vi "Initialize.vi"(8 "error in (no error)":errorcluster, 11 "State in":T1={"State"=enum."Idle", "Start Time"=timestamp(0 s since 1904-01-01), "Configuration"={"Cycle Period"=0.0, "Setpoint Entry"=0.0, "Output Device"=enum."Huber Ministat 230", "Huber Ministat 230 Settings"={"VISA resource name"="", "Simulated?"=FALSE}, "Lauda Settings"={"VISA resource name"="", "Simulated?"=FALSE, "Pump Power"=2}, "Julabo FP-50 Settings"={"VISA resource name"="", "Simulated?"=FALSE, "Pump Power"=2}, "Internal Control?"=FALSE, "Huber Unistat 410 Settings"={"VISA resource name"="", "Address"=0, "Simulated?"=FALSE}}, "Current Time"=timestamp(0 s since 1904-01-01), "First Iteration"=FALSE, "Data"={"TCU Speed"=0.0, "Temperature"=0.0}, "Process Name"="", "TCU On?"=FALSE, "Output Error"=FALSE, "Start Log"=FALSE, "Power Level Changed"=FALSE} {"Configuration"."Huber Unistat 410 Settings"."Address" min=0 max=99 format="%02.0f"; "Configuration"."Julabo FP-50 Settings"."Pump Power" min=0 max=8 step=1; "Configuration"."Lauda Settings"."Pump Power" min=0 max=8 step=1}) -> (0 "error out":errorcluster, 3 "State out":T1={"State"=enum."Idle", "Start Time"=timestamp(0 s since 1904-01-01), "Configuration"={"Cycle Period"=0.0, "Setpoint Entry"=0.0, "Output Device"=enum."Huber Ministat 230", "Huber Ministat 230 Settings"={"VISA resource name"="", "Simulated?"=FALSE}, "Lauda Settings"={"VISA resource name"="", "Simulated?"=FALSE, "Pump Power"=2}, "Julabo FP-50 Settings"={"VISA resource name"="", "Simulated?"=FALSE, "Pump Power"=2}, "Internal Control?"=FALSE, "Huber Unistat 410 Settings"={"VISA resource name"="", "Address"=0, "Simulated?"=FALSE}}, "Current Time"=timestamp(0 s since 1904-01-01), "First Iteration"=FALSE, "Data"={"TCU Speed"=0.0, "Temperature"=0.0}, "Process Name"="", "TCU On?"=FALSE, "Output Error"=FALSE, "Start Log"=FALSE, "Power Level Changed"=FALSE} {"Configuration"."Huber Unistat 410 Settings"."Address" min=0 max=99 format="%02.0f"; "Configuration"."Julabo FP-50 Settings"."Pump Power" min=0 max=8 step=1; "Configuration"."Lauda Settings"."Pump Power" min=0 max=8 step=1})   [LabVIEW 2018, in "TCU Module.lvlib" / "TCU Module Engine.lvlib"]
uses:
  TCU Module Engine.lvlib
  TCU State Cluster.ctl
  State Enum.ctl
  TCU Module Settings Cluster.ctl
  Output Devices.ctl
  Huber TCU/Huber Settings.ctl
  Lauda Integral XT-150 TCU/Lauda Settings.ctl
  Julabo Type 1 TCU/Julabo Type 1 TCU Folder/Julabo FP-50 Settings.ctl
  Huber Unistat 410 TCU/Huber Unistat 410 RS485 Settings.ctl
  Tag VIs/Tag FGV Operation Enum.ctl
  Shared Variables/Dynamic Shared Variables.lvlib
  Huber TCU/Huber Ministat 230 TCU.lvlib
  Lauda Integral XT-150 TCU/Lauda TCU.lvlib
  Julabo Type 1 TCU/Julabo Type 1 TCU Folder/Julabo Type FP-50 TCU.lvlib
  Huber Unistat 410 TCU/Huber Unistat 410 TCU.lvlib
  TCU Module.lvlib
panel:
  # "Output Instruments"
  # "Output Instruments"
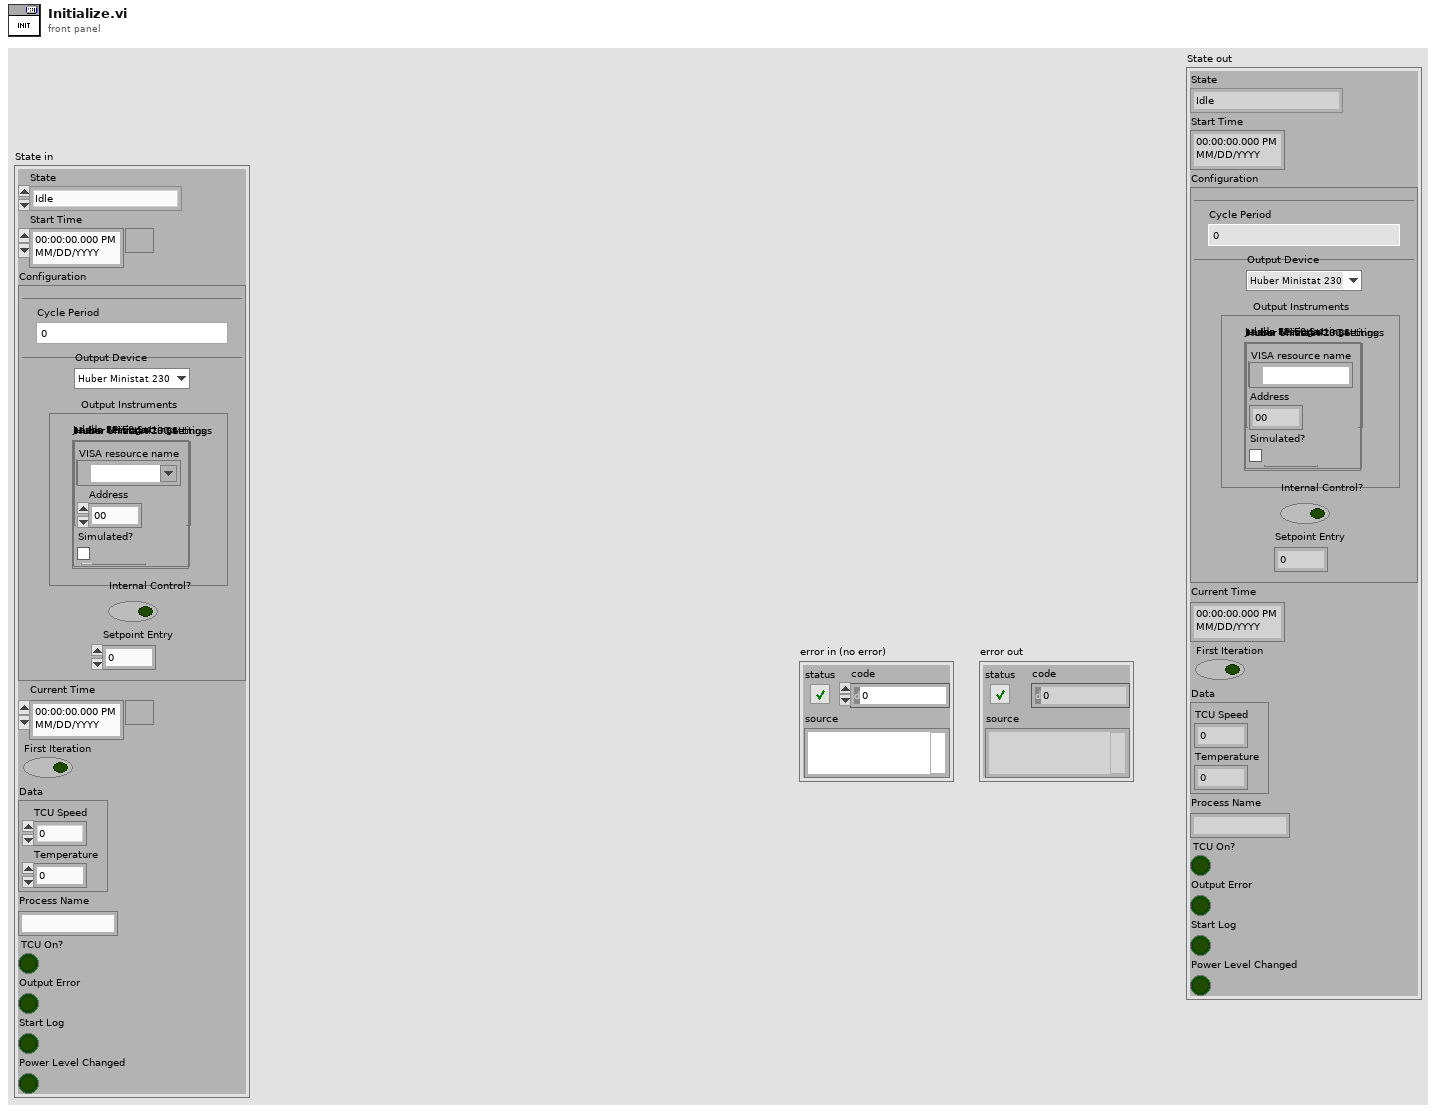
[diagram p1: front panel]
types:
  T1 = typedef "TCU Module.lvlib/TCU Module Engine.lvlib/TCU State Cluster.ctl" = cluster{"State":T2, "Start Time":timestamp, "Configuration":T3, "Current Time":timestamp, "First Iteration":bool, "Data":cluster{"TCU Speed":dbl, "Temperature":dbl}, "Process Name":string, "TCU On?":bool, "Output Error":bool, "Start Log":bool, "Power Level Changed":bool}
  T2 = typedef "TCU Module.lvlib/TCU Module Engine.lvlib/State Enum.ctl" = enum16{"Measuring", "Idle", "Paused"}
  T3 = typedef "TCU Module.lvlib/TCU Module Settings Cluster.ctl" = cluster{"Cycle Period":dbl, "Setpoint Entry":dbl, "Output Device":T4, "Huber Ministat 230 Settings":T5, "Lauda Settings":T6, "Julabo FP-50 Settings":T7, "Internal Control?":bool, "Huber Unistat 410 Settings":T8}
  T4 = typedef "Output Devices.ctl" = enum16{"Default", "Huber Ministat 230", "Huber Unistat 410", "Lauda XT-150", "Julabo FP-50"}
  T5 = typedef "Huber Ministat 230 TCU.lvlib/Huber Settings.ctl" = cluster{"VISA resource name":refnum<visa-resource-name>, "Simulated?":bool}
  T6 = typedef "Lauda TCU.lvlib/Lauda Settings.ctl" = cluster{"VISA resource name":refnum<visa-resource-name>, "Simulated?":bool, "Pump Power":i32}
  T7 = typedef "Julabo Type FP-50 TCU.lvlib/Julabo FP-50 Settings.ctl" = cluster{"VISA resource name":refnum<visa-resource-name>, "Simulated?":bool, "Pump Power":i32}
  T8 = typedef "Huber Unistat 410 TCU.lvlib/Huber Unistat 410 RS485 Settings.ctl" = cluster{"VISA resource name":refnum<visa-resource-name>, "Address":i8, "Simulated?":bool}
  T9 = typedef "Tag FGV Operation Enum.ctl" = enum16{"Init", "Set Notification Queue", "Create Tag", "Commit", "Write Tag (Numeric)", "Write Tag (Boolean)", "Read All Tags", "Read One Tag", "Delete Tag Category", "Set Alarm Parameters (Numeric)", "Set Alarm Parameters (Boolean)", "Enable All Alarms", "Disable All Alarms", "Delete All Tags", "Read Alarms", "Ack Alarm", "Read Alarm Parameters (Numeric)", "Read Alarm Parameters (Boolean)"}
  T10 = typedef "TCU Module.lvlib/TCU Module Tag Names Cluster.ctl" = cluster{"TCU Temp":string, "Output Device Tag":string, "TCU Speed":string, "Identifier Tag":string}
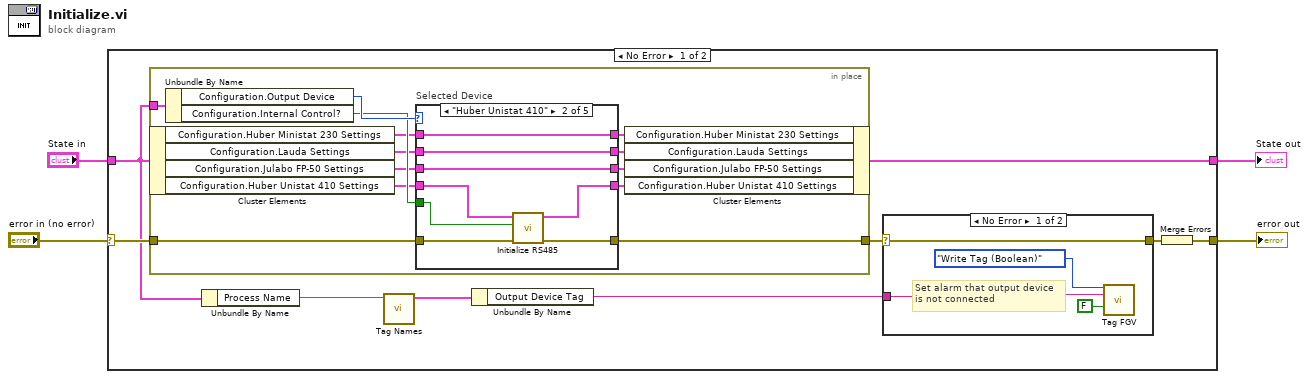
[diagram p0: block diagram]
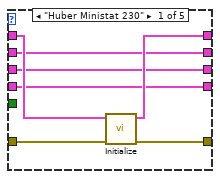
[diagram p2: hidden frame]
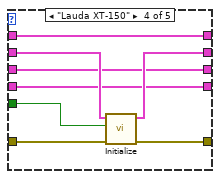
[diagram p4: hidden frame]
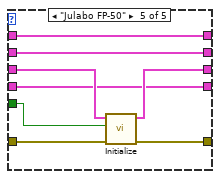
[diagram p5: hidden frame]
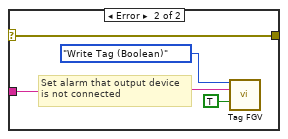
[diagram p6: hidden frame]
diagram:
  n1 = case shown="No Error" "error in (no error)" {
    selector: "error in (no error)" -> [w7 w72]
    tunnel: [w13 w72] -> w3
    tunnel: "State in" -> [w6 w71]
    tunnel: [w5 w71] -> w1
    frame No Error {
      n2 = in-place {
        in-place-border: w6 -> [w26]
        in-place-border: [w25] -> w12
        in-place-border: w7 -> [w23]
        n3 = in-place-cluster #1(w6) -> ("Configuration.Huber Ministat 230 Settings"=w21:T5, "Configuration.Lauda Settings"=w20:T6, "Configuration.Julabo FP-50 Settings"=w19:T7, "Configuration.Huber Unistat 410 Settings"=w18:T8)
        n4 = Unbundle By Name(w26) -> ("Configuration.Output Device"=w24:T4, "Configuration.Internal Control?"=w22:bool)
        n5 = case "Selected Device" shown="\"Huber Unistat 410\"" w24 {
          tunnel: w21 -> [w32 w39 w46 w50 w58]
          tunnel: [w33 w34 w44 w53 w61] -> w25
          tunnel: [w31 w39 w46 w50 w58] -> w17
          tunnel: w20 -> [w30 w40 w45 w51 w57]
          tunnel: [w30 w40 w45 w52 w57] -> w16
          tunnel: w23 -> [w29 w36 w44 w54 w62]
          tunnel: w19 -> [w28 w41 w43 w49 w60]
          tunnel: [w28 w41 w43 w49 w59] -> w15
          tunnel: w22 -> [_ w37 _ w48 w56]
          tunnel: w18 -> [w27 w38 w42 w47 w55]
          tunnel: [w27 w35 w42 w47 w55] -> w14
          frame "Huber Ministat 230" {
            n6 = call "Initialize.vi"("error in (no error)"=w29, "Huber Settings"=w32) -> ("error out"=w33:errorcluster, "Huber Settings"=w31:T5)  [unwired: 7 in, 1 out]
          }
          frame "Huber Unistat 410" {
            n7 = call "Initialize RS485.vi"("error in (no error)"=w36, "Internal?"=w37, "Huber Unistat 410 Settings"=w38) -> ("error out"=w34:errorcluster, "Huber Unistat 410 Settings 2"=w35:T8)  [unwired: 6 in, 1 out]
          }
          frame "Default", Default {
          }
          frame "Lauda XT-150" {
            n8 = call "Initialize.vi"("error in (no error)"=w54, "Internal?"=w48, "Lauda Settings In"=w51) -> ("error out"=w53:errorcluster, "Lauda Settings Out"=w52:T6)  [unwired: 6 in, 1 out]
          }
          frame "Julabo FP-50" {
            n9 = call "Initialize.vi"("error in (no error)"=w62, "Internal?"=w56, "Julabo FP-50 Settings"=w60) -> ("error out"=w61:errorcluster, "Julabo FP-50 Settings"=w59:T7)  [unwired: 6 in, 1 out]
          }
        }
        n10 = in-place-cluster #1("Configuration.Huber Ministat 230 Settings"=w17, "Configuration.Lauda Settings"=w16, "Configuration.Julabo FP-50 Settings"=w15, "Configuration.Huber Unistat 410 Settings"=w14) -> (w5:T1)
      }
      n11 = Unbundle By Name(w6) -> ("Process Name"=w9:string)
      n12 = call "Tag Names.vi"("Process Name"=w9) -> ("Pump Module Tag Names"=w8:T10)  [unwired: 8 in, 2 out]
      n13 = Unbundle By Name(w8) -> ("Output Device Tag"=w10:string)
      n14 = case shown="No Error" w12 {
        selector: w12 -> [w66 w70]
        tunnel: [w66 w70] -> w11
        tunnel: w10 -> [w63 w69]
        frame No Error {
          # "Set alarm that output device\nis not connected"
          n15 = call "Tag FGV.vi"("Operation"=Tag_FGV_Operation_Enum."Write Tag (Boolean)", "Tag Name"=w63, "Data"=FALSE) -> ()  [unwired: 5 in, 8 out]
        }
        frame Error {
          # "Set alarm that output device\nis not connected"
          n16 = call "Tag FGV.vi"("Operation"=Tag_FGV_Operation_Enum."Write Tag (Boolean)", "Tag Name"=w69, "Data"=TRUE) -> ()  [unwired: 5 in, 8 out]
        }
      }
      n17 = Merge Errors(w11) -> (w13:errorcluster)
    }
    frame Error {
    }
  }
  "error out" <- w3
  "State out" <- w1
